vi "To Multibyte string_DK.vi"(3 "error in":errorcluster, 4 "Big Endian?":bool, 5 "Code Page":i32(ring) items=["System default"=0, "Latin-1"=1252, "Japanese"=932, "Korean"=947, "Chinese simplified"=936, "Chinese traditional"=950, "Central Europe"=1250, "Cyrillic"=1251, "Greek"=1253, "Turkish"=1254, "Hebrew"=1255, "Arabic"=1256, "Baltic"=1257, "Thai"=874, "Vietnamese"=783, "UTF8"=65001, "UTF-7"=65000], 6 "Unicode String":string="t\u0000é\u0000t\u0000é\u0000") -> (0 "error out":errorcluster, 2 "Multibyte string":string="tété")   [LabVIEW 2024]
uses:
  kernel32.dll
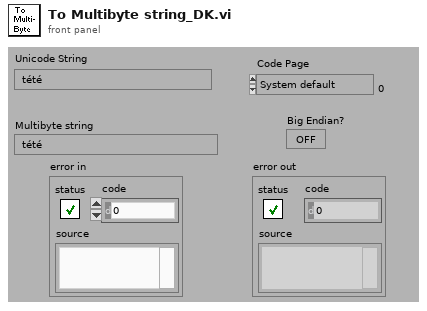
[diagram p1: front panel]
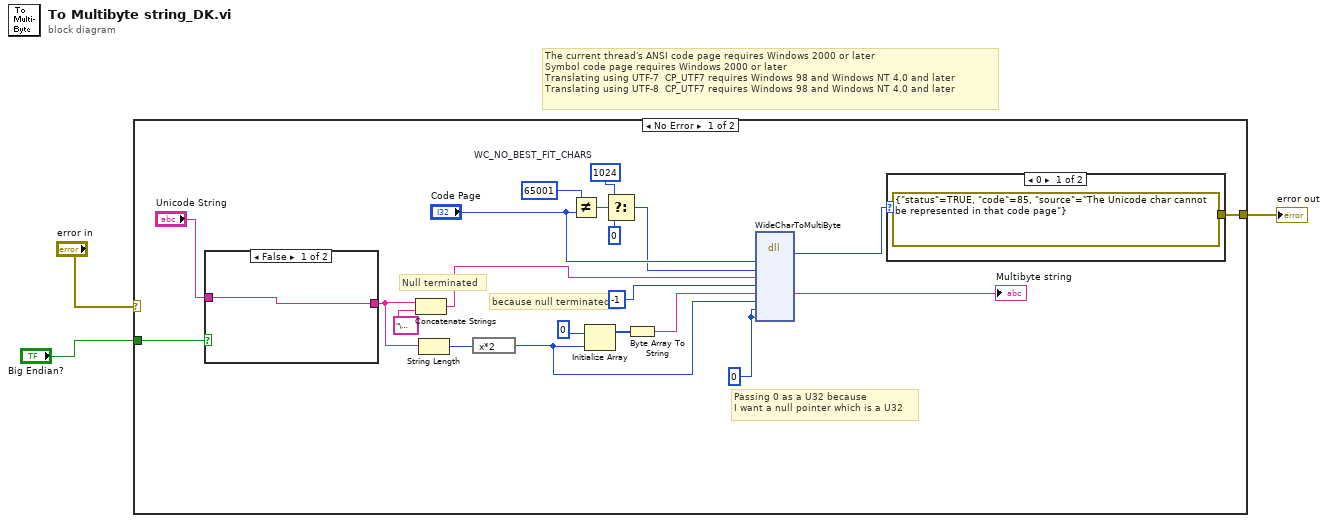
[diagram p0: block diagram]
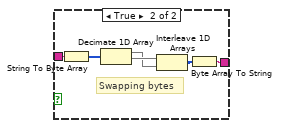
[diagram p2: hidden frame]
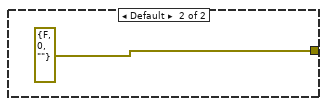
[diagram p3: hidden frame]
diagram:
  # "The current thread's ANSI code page requires Windows 2000 or later\nSymbol code page requires Windows 2000 or later\nTranslating using UTF-7  CP_UTF7 requires Windows 98 and Windows NT 4.0 and later\nTranslating using UTF-8  CP_UTF7 requires Windows 98 and Windows NT 4.0 and later"
  n1 = case shown="No Error" "error in" {
    selector: "error in" -> [_ w34]
    tunnel: [w5 w34] -> w3
    tunnel: "Big Endian?" -> [w4 _]
    frame No Error {
      w7 = u32 0 ("usedefault")
      w22 = u32 1024  # WC_NO_BEST_FIT_CHARS
      # "Passing 0 as a U32 because\nI want a null pointer which is a U32"
      # "because null terminated"
      # "Null terminated"
      n2 = case shown="False" w4 {
        tunnel: "Unicode String" -> [w25 w27]
        tunnel: [w25 w26] -> w10
        frame False {
        }
        frame True {
          # "Swapping bytes"
          n3 = String To Byte Array(string=w27) -> (unsigned byte array=w28:u8[])
          n4 = Decimate 1D Array(w28) -> (w30:u8[], w31:u8[])
          n5 = Interleave 1D Arrays(w31, w30) -> (w29:u8[])
          n6 = Byte Array To String(unsigned byte array=w29) -> (string=w26:string)
        }
      }
      n7 = Concatenate Strings(w10, "\u0000" ("chaîne")) -> (w14:string)
      n8 = String Length(string=w10) -> (length=w12:i32)
      n9 = expression code="x*2"(w12) -> (w9:i32)
      n10 = Not Equal?(x=u32 65001, y="Code Page") -> (x != y?=w23:bool)
      n11 = Initialize Array(u8 0, w9) -> (w18:u8[])
      n12 = Select(t=w22, s=w23, f=u32 0) -> (s? t:f=w8:u32)
      n13 = Byte Array To String(unsigned byte array=w18) -> (string=w17:string)
      n14 = dll-call lib="Kernel32.DLL" fn="WideCharToMultiByte"("Codepage"="Code Page", "dwFlags"=w8, "widestring"=w14, "nbchar"=-1, "buffernewstring"=w17, "buffersize"=w9, "defaultchar"=w7, "usedefault"=w7) -> (w6:i32, "buffernewstring"=→"Multibyte string":string)  [unwired: 10 in, 2 out]
      n15 = case shown="0" w6 {
        tunnel: [errorcluster {"status"=TRUE, "code"=85, "source"="The Unicode char cannot be represented in that code page"} ("error out") errorcluster {"status"=FALSE, "code"=0, "source"=""} ("error out")] -> w5
        frame 0 {
        }
        frame Default {
        }
      }
    }
    frame Error {
    }
  }
  "error out" <- w3
